vi "SetVoltage.vi"(8 "error in (no error)":errorcluster, 10 "Voltage":dbl, 11 "Multiplexer_Opmux in":refnum<class "Multiplexer_Opmux.lvclass">) -> (0 "error out":errorcluster, 3 "Multiplexer_Opmux out":refnum<class "Multiplexer_Opmux.lvclass">)   [LabVIEW 2013, in "Multiplexer_Opmux.lvclass"]
uses:
  Multiplexer_Opmux.lvclass
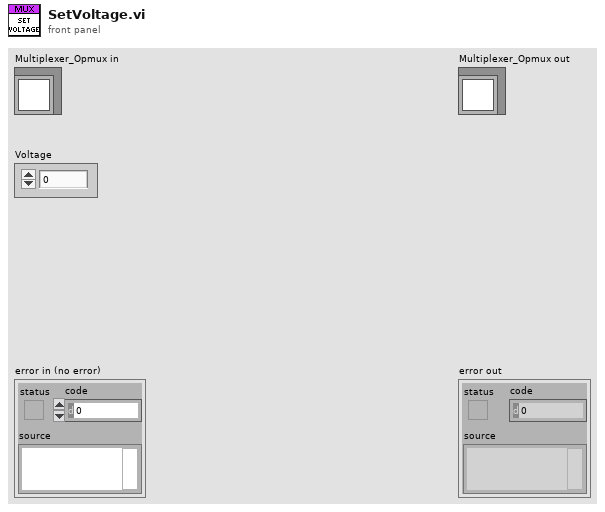
[diagram p1: front panel]
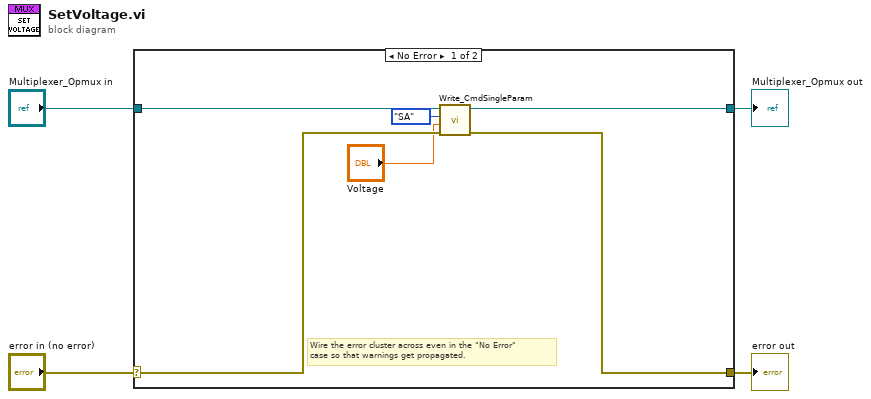
[diagram p0: block diagram]
diagram:
  n1 = case shown="No Error" "error in (no error)" {
    selector: "error in (no error)" -> [w7 w12]
    tunnel: [w6 w12] -> w3
    tunnel: [w9 w11] -> w1
    tunnel: "Multiplexer_Opmux in" -> [w10 w11]
    frame No Error {
      # "Wire the error cluster across even in the \"No Error\"\ncase so that warnings get propagated."
      n2 = call-dynamic "Write_CmdSingleParam.vi"("error in (no error)"=w7, "Param"="Voltage", "Command"=enum16{"SA", "GT", "SI", "SL", "ST", "CT"}."SA", "Multiplexer_Opmux in"=w10) -> ("error out"=w6:errorcluster, "Multiplexer_Opmux out"=w9:refnum<class "Multiplexer_Opmux.lvclass">)  [unwired: 6 in]
    }
    frame Error {
    }
  }
  "error out" <- w3
  "Multiplexer_Opmux out" <- w1
